vi "CreatePoly.vi"   [LabVIEW 2020]
uses:
  g_ar_toolkit.capture/CameraStream/CameraStream.lvclass
  <vilib>/Utility/miscctls.llb/LVMapReplaceAction.ctl
  269c9377-1933-43b6-923f-e4fc9fbce505.vi
  <vilib>/Comparison/Equal/Equal Functor/Equal Functor.lvclass
  <vilib>/regexp/Match Regular Expression.xnode
types:
  T1 = typedef "LVMapReplaceAction.ctl" = enum32{"Modify Entry only if found", "Add or Modify Entry", "Delete Entry"}
  T2 = enum32{"invalid VI type", "Standard VI", "Control VI", "Global VI", "Polymorphic VI", "Configuration VI", "SubSystem", "Facade VI", "Method VI", "Statechart Diagram VI"}
  T3 = cluster{"VIPath":path, "Menu Name":string, "Selector Name":string}
  T4 = cluster{"VIPath":path, "Menu Name":string, "Selector Name":string}[]
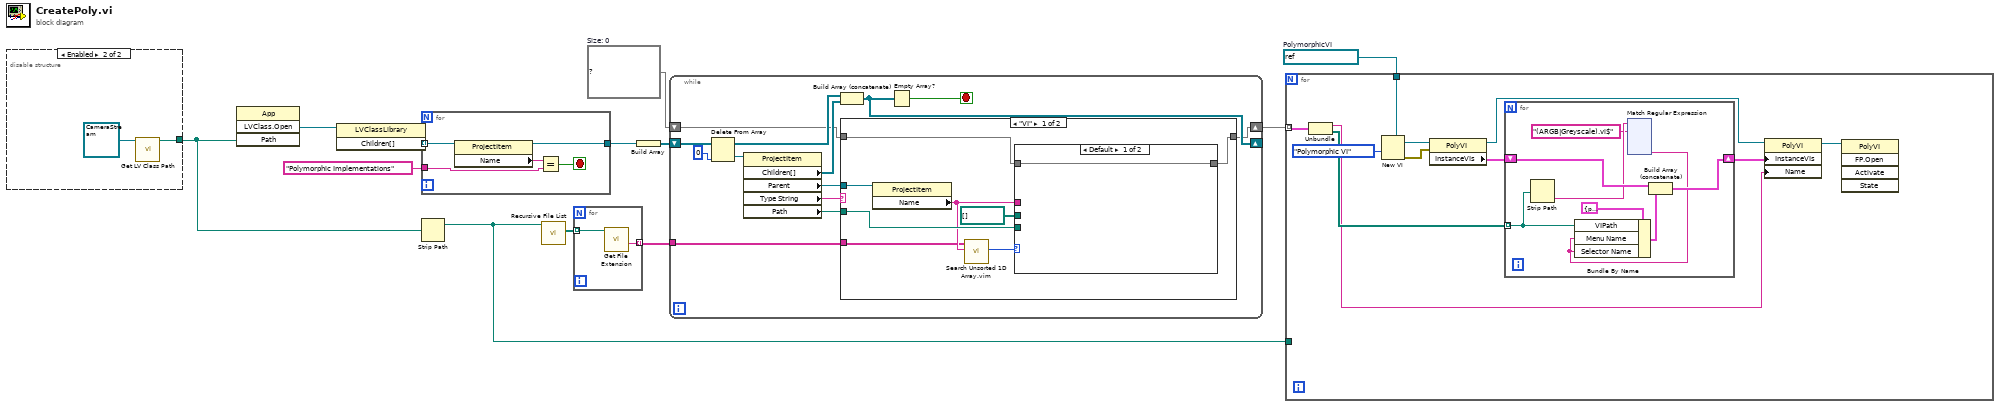
[diagram p0: block diagram]
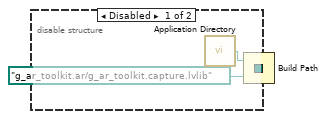
[diagram p2: hidden frame]
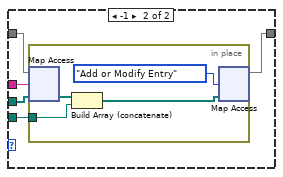
[diagram p3: hidden frame]
diagram:
  w1 = refnum<vi> refnum  # PolymorphicVI
  w7 = map{string, path[]} {}  # Size: 0
  n1 = disable-structure shown="Enabled" {
    disable-tunnel: [w14 w16] -> w6
    frame Disabled {
      n2 = call <vilib>:"Application Directory.vi"() -> ("Application Directory"=w15:path)
      n3 = Build Path(base path=w15, name or relative path=path "g_ar_toolkit.ar/g_ar_toolkit.capture.lvlib" ("Path")) -> (appended path=w14:path)
    }
    frame Enabled {
      n4 = call <vilib>:"Get LV Class Path.vi"("object"=refnum<class "CameraStream.lvclass"> refnum ("g_ar_toolkit.capture.lvlib:CameraStream.lvclass")) -> ("class path"=w16:path)  [unwired: 9 in, 1 out]
    }
  }
  n5 = invoke class="App" method="LVClass.Open"("Path"=w6) -> ("LVClass.Open"=w12:refnum<vi>)  [unwired: 3 in, 3 out]
  n6 = property class="LVClassLibrary"(reference=w12) -> ("Children[]"=w11:refnum<vi>[])  [unwired: 1 in, 2 out]
  n7 = for {
    tunnel: w11 -> [w22] mode=indexing
    tunnel: [w21] -> w10
    tunnel: "Polymorphic Implementations" ("y") -> [w19]
    stop <- w18 stop-if-true
    n8 = property class="ProjectItem"(reference=w22) -> (reference out=w21:refnum<vi>, "Name"=w20:string)  [unwired: 1 in, 1 out]
    n9 = Equal?(x=w20, y=w19) -> (x = y?=w18:bool)
  }
  n10 = Strip Path(path=w6) -> (stripped path=w2:path)  [unwired: 1 out]
  n11 = call <vilib>:"Recursive File List.vi"("Folder Path"=w2) -> ("All Files in Dir"=w5:path[])  [unwired: 6 in, 4 out]
  n12 = for {
    tunnel: w5 -> [w24] mode=indexing
    tunnel: [w23] -> w4 mode=indexing
    n13 = call <vilib>:"Get File Extension.vi"("file"=w24) -> ("filename without extension"=w23:string)  [unwired: 6 in, 4 out]
  }
  n14 = Build Array(w10) -> (w9:refnum<vi>[])
  n15 = while {
    shift-right: [w33] -> _
    shift-left: w9 -> [w37]
    shift-right: [w27] -> w3
    shift-left: w7 -> [w26]
    tunnel: w4 -> [w25]
    stop <- w32 stop-if-true
    n16 = Delete From Array(array=w37, index=0) -> (deleted portion=w35:refnum<vi>, array with subset deleted=w34:refnum<vi>[])  [unwired: 1 in]
    n17 = property class="ProjectItem"(reference=w35) -> ("Children[]"=w30:refnum<vi>[], "Parent"=w29:refnum<vi>, "Type String"=w31:string, "Path"=w28:path)  [unwired: 1 in, 2 out]
    n18 = Build Array (concatenate)(w34, w30) -> (w33:refnum<vi>[])
    n19 = case shown="\"VI\"" w31 {
      tunnel: w29 -> [w45 _]
      tunnel: w28 -> [w43 _]
      tunnel: [w42 w56] -> w27
      tunnel: w26 -> [w41 w56]
      tunnel: w25 -> [w39 _]
      frame "VI" {
        n20 = property class="ProjectItem"(reference=w45) -> ("Name"=w40:string)  [unwired: 1 in, 2 out]
        n21 = call "Search Unsorted 1D Array.vim"("element"=w40, "unsorted 1D array"=w39) -> ("index of element"=w38:i32)  [unwired: 9 in]
        n22 = case shown="Default" w38 {
          tunnel: path[] [] -> [_ w51]
          tunnel: w43 -> [_ w50]
          tunnel: [w46 w49] -> w42
          tunnel: w41 -> [w46 w48]
          tunnel: w40 -> [_ w47]
          frame Default {
          }
          frame -1 {
            n23 = in-place {
              in-place-border: w50 -> [w54]
              n24 = in-place-map #1(w48, w47, w51) -> (w55:path[])  [unwired: 1 out]
              n25 = Build Array (concatenate)(w55, w54) -> (w53:path[])
              n26 = in-place-map #1(w53, LVMapReplaceAction."Add or Modify Entry" ("action")) -> (w49:map{string, path[]})  [unwired: 2 out]
            }
          }
        }
      }
      frame Default {
      }
    }
    n27 = Empty Array?(array=w33) -> (empty?=w32:bool)
  }
  n28 = for {
    tunnel: w3 -> [w67] mode=indexing
    tunnel: w1 -> [w66]
    tunnel: w2 -> [_]
    n29 = Unbundle(w67) -> ("Name"=w59:string, w62:path[])
    n30 = New VI(5:w66, 9:T2."Polymorphic VI" ("vi type (standard vi)")) -> (0:w64:errorcluster, 3:w65:refnum<vi>)  [unwired: 5 in]
    n31 = property class="PolyVI"(reference=w65, error in=w64) -> (reference out=w60:refnum<vi>, "InstanceVIs"=w63:T4)  [unwired: 1 out]
    n32 = for {
      shift-right: [w74] -> w61
      shift-left: w63 -> [w75]
      tunnel: w62 -> [w71] mode=indexing
      n33 = Strip Path(path=w71) -> (name=w70:string)  [unwired: 1 out]
      n34 = xnode "Match Regular Expression"("input string"=w70, "regular expression"="(ARGB|Greyscale).vi$") -> ("submatch 1"=w68:string)  [unwired: 4 in, 5 out]
      n35 = Bundle By Name(cluster=T3 {"VIPath"=path "", "Menu Name"="", "Selector Name"=""}, "VIPath"=w71, "Menu Name"=w68, "Selector Name"=w68) -> (w72:T3)
      n36 = Build Array (concatenate)(w75, w72) -> (w74:T4)
    }
    n37 = property class="PolyVI"(reference=w60, "InstanceVIs"=w61, "Name"=w59) -> (reference out=w58:refnum<vi>)  [unwired: 1 in, 1 out]
    n38 = invoke class="PolyVI" method="FP.Open"(reference=w58) -> ()  [unwired: 4 in, 5 out]
  }
